vi "SearchStringPattern.vi"(2 "Pattern To Search":string, 3 "String To Search":string) -> (0 "Offset Past Match":i32, 1 "String Found?":bool)   [LabVIEW 2021]
doc: "This Vi will search a string for a pattern. If the pattern is detected it returns a true boolean and the FIRST index of the pattern. If it is not it returns a false boolean and an offset of -1."
panel:
  out "The Change":string
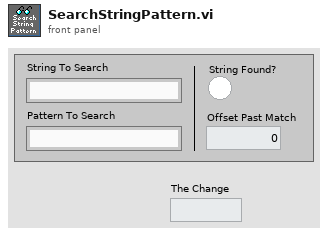
[diagram p1: front panel]
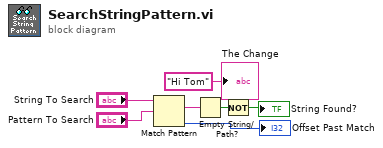
[diagram p0: block diagram]
diagram:
  n1 = Match Pattern(string="String To Search", regular expression="Pattern To Search") -> (match substring=w5:string, offset past match=→"Offset Past Match":i32)  [unwired: 1 in, 2 out]
  n2 = Empty String/Path?(string/path=w5) -> (empty?=w3:bool)
  n3 = Not(x=w3) -> (.not. x?=→"String Found?":bool)
  "The Change" <- "Hi Tom" ("The Change")
